vi "Axis modifications.vi"(1 "Driver JoyStick Info":T2) -> (0 "Driver JoyStick Info 2":T2)   [LabVIEW 2012]
uses:
  <vilib>/Rock Robotics/WPI/Solenoid/WPI_SolenoidValue.ctl
  Drive Global Data.vi
panel:
  # "X"
  # "Y"
  # "X"
  # "Y"
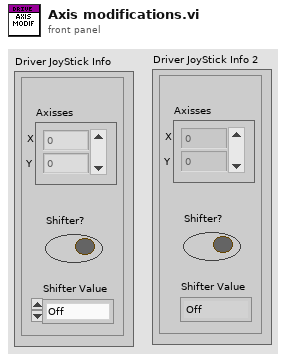
[diagram p1: front panel]
types:
  T1 = typedef "WPI_SolenoidValue.ctl" = enum16{"Off", "On", "Forward", "Reverse"}
  T2 = cluster{"Shifter?":bool, "Axisses":dbl[], "Shifter Value":T1}
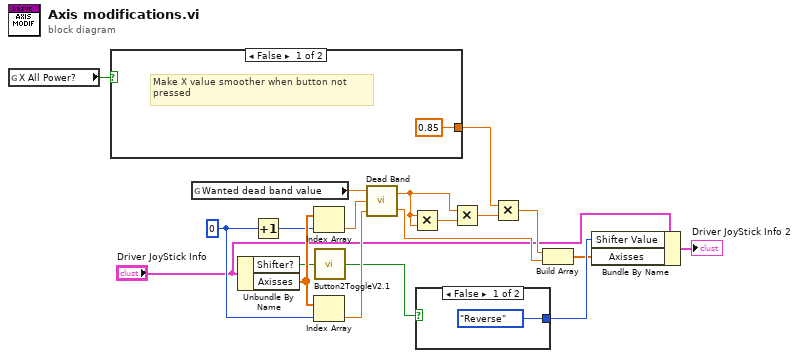
[diagram p0: block diagram]
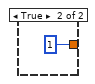
[diagram p2: hidden frame]
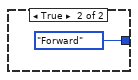
[diagram p3: hidden frame]
diagram:
  w17 = 0 ("index")
  n1 = global read "Drive Global Data.vi" "X All Power?"() -> (w10:bool)
  n2 = case shown="False" w10 {
    tunnel: [0.85 1] -> w11
    frame False {
      # "Make X value smoother when button not \npressed"
    }
    frame True {
    }
  }
  n3 = global read "Drive Global Data.vi" "Wanted dead band value"() -> (w14:dbl)
  n4 = Unbundle By Name("Driver JoyStick Info") -> ("Shifter?"=w2:bool, "Axisses"=w19:dbl[])
  n5 = Increment(x=w17) -> (x+1=w18:i32)
  n6 = Index Array(array=w19, index=w18) -> (element=w13:dbl)
  n7 = Index Array(array=w19, index=w17) -> (element=w12:dbl)
  n8 = call "Button2ToggleV2.1.vi"("a"=w2) -> ("Result(clone)"=w1:bool)
  n9 = call "Dead Band.vi"("Axis 2 In"=w12, "Axis 1 In"=w13, "Dead Band"=w14) -> ("Axis 2 Out"=w15:dbl, "Axis 1 Out"=w8:dbl)
  n10 = Multiply(x=w8, y=w8) -> (x*y=w9:dbl)
  n11 = case shown="False" w1 {
    tunnel: [WPI_SolenoidValue."Reverse" ("Value") WPI_SolenoidValue."Forward" ("Value")] -> w4
    frame False {
    }
    frame True {
    }
  }
  n12 = Multiply(x=w8, y=w9) -> (x*y=w7:dbl)
  n13 = Multiply(x=w11, y=w7) -> (x*y=w16:dbl)
  n14 = Build Array(w16, w15) -> (w3:dbl[])
  n15 = Bundle By Name(cluster="Driver JoyStick Info", "Shifter Value"=w4, "Axisses"=w3) -> (→"Driver JoyStick Info 2":T2)
